vi "CloseSink.vi"(8 "error in (no error)":errorcluster, 11 "FileAppender in":refnum<class "FileAppender.lvclass">) -> (0 "error out":errorcluster, 3 "FileAppender out":refnum<class "FileAppender.lvclass">)   [LabVIEW 2026, in "Lumberjack.lvlib" / "FileAppender.lvclass"]
doc: "Flush and close this appender's sink resource. Called once on actor exit (from Actor Core), including the error-exit path, so buffered data is not lost on shutdown. Abstract: each concrete appender closes its own sink. DD, must override."
uses:
  FileAppender.lvclass
  FileAppender.lvclass/FileAppender.ctl
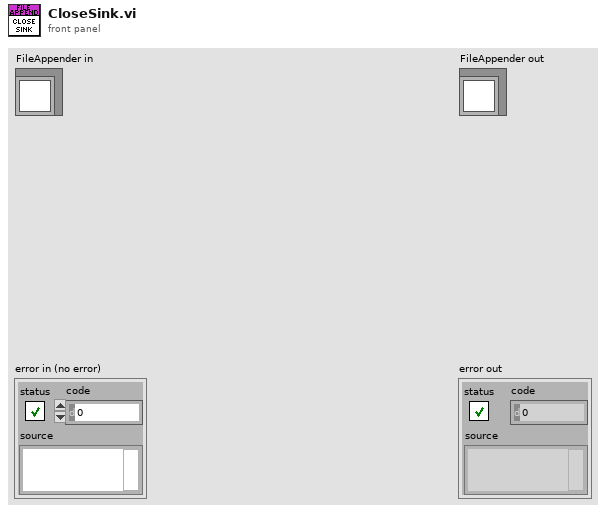
[diagram p1: front panel]
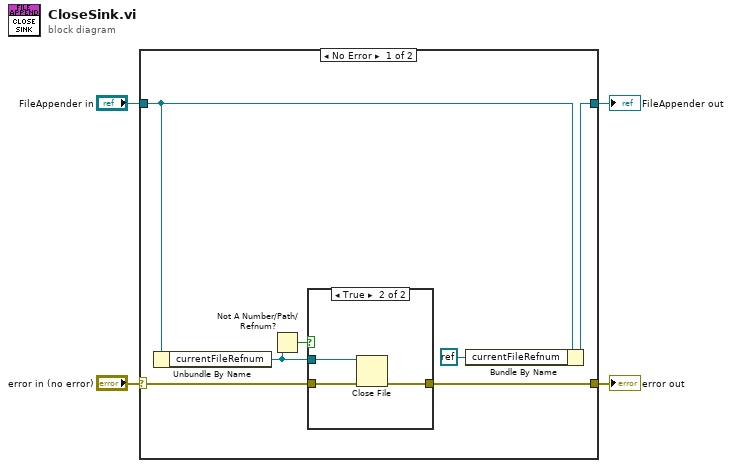
[diagram p0: block diagram]
diagram:
  n1 = case shown="No Error" "error in (no error)" {
    selector: "error in (no error)" -> [w11 w17]
    tunnel: [w10 w17] -> w4
    tunnel: [w6 w16] -> w3
    tunnel: "FileAppender in" -> [w7 w16]
    frame No Error {
      n2 = Unbundle By Name(w7) -> ("currentFileRefnum"=w9:refnum<file>)
      n3 = Not A Number/Path/Refnum?(number/path/refnum=w9) -> (NaN/Path/Refnum?=w8:bool)
      n4 = case shown="True" w8 {
        tunnel: w9 -> [_ w15]
        tunnel: w11 -> [w12 w14]
        tunnel: [w12 w13] -> w10
        frame False {
        }
        frame True {
          n5 = Close File(refnum=w15, error in=w14) -> (error out=w13:errorcluster)  [unwired: 1 out]
        }
      }
      n6 = Bundle By Name(cluster=w7, "currentFileRefnum"=refnum<k0> refnum) -> (w6:refnum<class "FileAppender.lvclass">)
    }
    frame Error {
    }
  }
  "error out" <- w4
  "FileAppender out" <- w3
